vi "FPGA Read All FIFO Address by Index.vi"(8 "error in (no error)":errorcluster, 9 "index":i32, 11 "FPGA Interface Base in":refnum<class "FPGA Interface Base.lvclass">) -> (0 "error out":errorcluster, 1 "Found?":bool, 2 "Address":u32, 3 "FPGA Interface Base out":refnum<class "FPGA Interface Base.lvclass">)   [LabVIEW 2010, in "FPGA Interface Base.lvclass"]
uses:
  <userlib>/_FPGA Interface Advanced Tools/FPGA Interface Base/FPGA Interface Base.lvclass
  <userlib>/_FPGA Interface Advanced Tools/FPGA Interface Base/FPGA Interface Base.lvclass/FPGA Interface Base.ctl
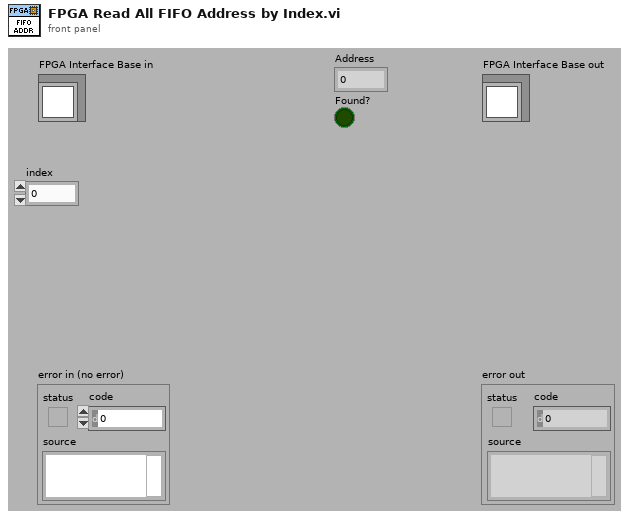
[diagram p1: front panel]
types:
  T1 = typedef "FPGA Interface Base.lvclass/FPGA Session.ctl" = refnum<data-value>
  T2 = typedef "FPGA Interface Base.lvclass/FPGA Session Data.ctl" = cluster{"Session Out":u32, "Indicator Scalars":T3, "Indicator Arrays":T5, "Control Scalars":T3, "Control Arrays":T5, "TargetToHost FIFO Channels":T7, "HostToTarget FIFO Channels":T7, "All FIFOs":T8[], "IRQ Context Queue":refnum<queue>}
  T3 = typedef "FPGA Bitfile Utility.lvlib/Scalar Register Set.ctl" = cluster{"Boolean":T4[], "I8":T4[], "I16":T4[], "I32":T4[], "I64":T4[], "U8":T4[], "U16":T4[], "U32":T4[], "U64":T4[]}
  T4 = typedef "FPGA Bitfile Utility.lvlib/Scalar Register.ctl" = cluster{"Address":u32, "Name":string}
  T5 = typedef "FPGA Bitfile Utility.lvlib/Array Register Set.ctl" = cluster{"Boolean":T6[], "I8":T6[], "I16":T6[], "I32":T6[], "I64":T6[], "U8":T6[], "U16":T6[], "U32":T6[], "U64":T6[]}
  T6 = typedef "FPGA Bitfile Utility.lvlib/Array Register.ctl" = cluster{"Address":u32, "Num Elements":u32, "Name":string}
  T7 = typedef "FPGA Bitfile Utility.lvlib/FIFO Channel Set.ctl" = cluster{"Boolean":T8[], "I8":T8[], "I16":T8[], "I32":T8[], "I64":T8[], "U8":T8[], "U16":T8[], "U32":T8[], "U64":T8[]}
  T8 = typedef "FPGA Bitfile Utility.lvlib/FIFO Channel.ctl" = cluster{"Physical Channel":u32, "Name":string}
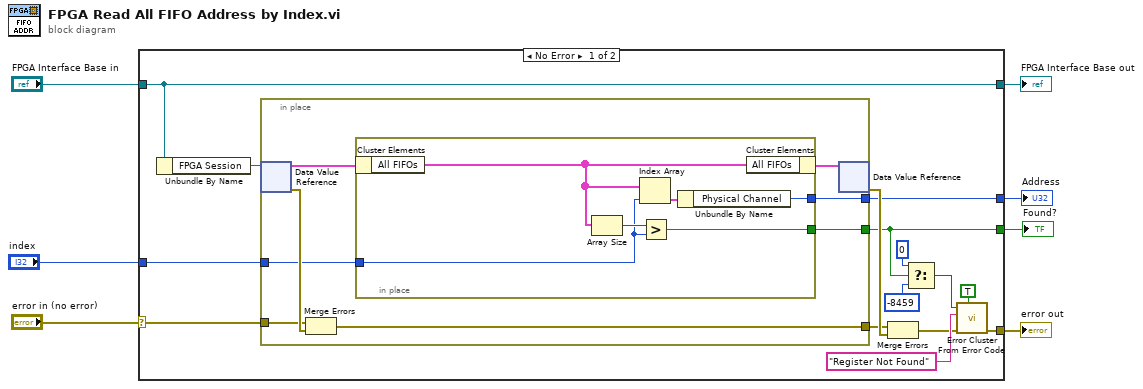
[diagram p0: block diagram]
diagram:
  n1 = case shown="No Error" "error in (no error)" {
    selector: "error in (no error)" -> [w17 w37]
    tunnel: [w9 w37] -> w6
    tunnel: [w22 w38] -> w4
    tunnel: "FPGA Interface Base in" -> [w22 w38]
    tunnel: [w18 _] -> w3
    tunnel: [w8 _] -> w2
    tunnel: "index" -> [w16 _]
    frame No Error {
      n2 = Unbundle By Name(w22) -> ("FPGA Session"=w19:T1)
      n3 = in-place {
        in-place-border: [w27] -> w18
        in-place-border: [w26] -> w8
        in-place-border: [w25] -> w20
        in-place-border: w17 -> [w24]
        in-place-border: w16 -> [w23]
        n4 = in-place-dvr #1(w19) -> (w29:T2, w30:errorcluster)
        n5 = Merge Errors(w24, w30) -> (w25:errorcluster)
        n6 = in-place {
          in-place-border: [w36] -> w27
          in-place-border: [w34] -> w26
          in-place-border: w23 -> [w31]
          n7 = in-place-cluster #2(w29) -> ("All FIFOs"=w33:T8[])
          n8 = Array Size(array=w33) -> (size(s)=w35:i32)
          n9 = Index Array(array=w33, index=w31) -> (element=w32:T8)
          n10 = Greater?(x=w35, y=w31) -> (0:w34:bool)
          n11 = Unbundle By Name(w32) -> ("Physical Channel"=w36:u32)
          n12 = in-place-cluster #2("All FIFOs"=w33) -> (w28:T2)
        }
        n13 = in-place-dvr #1(w28) -> (w21:errorcluster)  [unwired: 1 out]
      }
      n14 = Merge Errors(w20, w21) -> (w10:errorcluster)
      n15 = Select(t=0, s=w8, f=-8459 ("error code (0)")) -> (s? t:f=w14:i32)
      n16 = call <vilib>:"Error Cluster From Error Code.vi"("show call chain? (False)"=TRUE, "error in (no error)"=w10, "error message (\"\")"="Register Not Found" ("string"), "error code (0)"=w14) -> ("error out"=w9:errorcluster)  [unwired: 5 in]
    }
    frame Error {
    }
  }
  "error out" <- w6
  "FPGA Interface Base out" <- w4
  "Address" <- w3
  "Found?" <- w2
